vi "FindPressure.vi"(0 "Pressure Calc":u16(ring)=1 items=["Pos Peak", "Neg peak", "Pk-Pk", "Steady State", "CW Drive", "Pii"], 1 "time step (s)":sgl=1e-10 format="%.2e", 3 "Input":dbl[][](array[numeric]) format="%.2f") -> (5 "Pressures":dbl[](array[numeric]) format="%.2f")   [LabVIEW 2022 SP3]
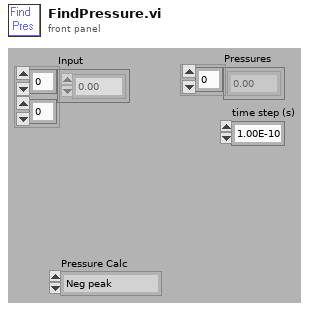
[diagram p1: front panel]
types:
  T1 = cluster{"Frequency (MHz)":dbl, "prf":dbl, "focal length (cm)":dbl, "derating (.3) factor":dbl, "neg peak pressure (MPa)":dbl, "pos peak pressure (MPa)":dbl, "p.3":dbl, "pulse dur (Pd s)":dbl, "Pulse Int \nIntegral (PII J/cm^2)":dbl, "Pulse Av Intensity\n (Ipa W/cm^2)":dbl, "Ipa.3":dbl, "Temporal Av Intensity \n(Ita mW/cm^2)":dbl, "Ita.3":dbl, "MI":dbl}
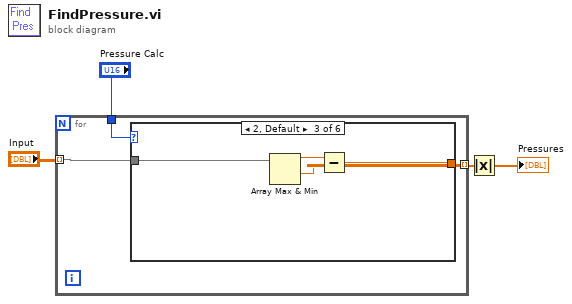
[diagram p0: block diagram]
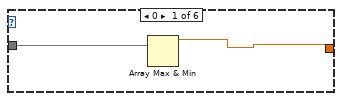
[diagram p2: hidden frame]
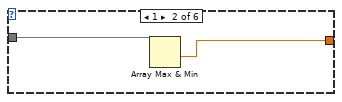
[diagram p3: hidden frame]
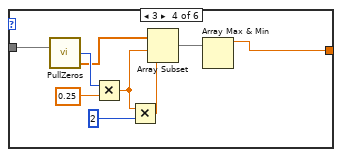
[diagram p4: hidden frame]
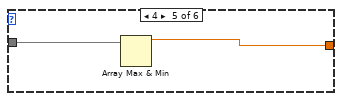
[diagram p5: hidden frame]
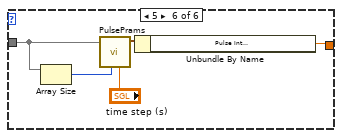
[diagram p6: hidden frame]
diagram:
  n1 = for {
    tunnel: "Input" -> [w6] mode=indexing
    tunnel: [w5] -> w3 mode=indexing
    tunnel: "Pressure Calc" -> [w7]
    n2 = case shown="2, Default" w7 {
      tunnel: w6 -> [w9 w11 w15 w18 w26 w28]
      tunnel: [w8 w10 w12 w16 w25 w30] -> w5
      frame 0 {
        n3 = Array Max & Min(array=w9) -> (max value=w8:dbl)  [unwired: 3 out]
      }
      frame 1 {
        n4 = Array Max & Min(array=w11) -> (min value=w10:dbl)  [unwired: 3 out]
      }
      frame 2, Default {
        n5 = Array Max & Min(array=w15) -> (max value=w14:dbl, min value=w13:dbl)  [unwired: 2 out]
        n6 = Subtract(x=w14, y=w13) -> (x-y=w12:dbl)
      }
      frame 3 {
        n7 = call "PullZeros.vi"("input"=w18) -> ("output"=w19:dbl[], "non zero points"=w22:i32)  [unwired: 3 out]
        n8 = Multiply(x=w22, y=0.25) -> (x*y=w24:dbl)
        n9 = Multiply(x=w24, y=2) -> (x*y=w21:dbl)
        n10 = Array Subset(array=w19, index=w24, length=w21) -> (w17:dbl[])
        n11 = Array Max & Min(array=w17) -> (max value=w16:dbl)  [unwired: 3 out]
      }
      frame 4 {
        n12 = Array Max & Min(array=w26) -> (max value=w25:dbl)  [unwired: 3 out]
      }
      frame 5 {
        n13 = Array Size(array=w28) -> (size(s)=w27:i32)
        n14 = call "PulsePrams.vi"("sample rate (s/Pt)"="time step (s)", "Length of Subset"=w27, "Data"=w28) -> ("Pulse Parameters"=w31:T1)  [unwired: 4 in, 4 out]
        n15 = Unbundle By Name(w31) -> ("Pulse Int \nIntegral (PII J/cm^2)"=w30:dbl)
      }
    }
  }
  n16 = Absolute Value(x=w3) -> (abs(x)=→"Pressures":dbl[])
